vi "PVreader.vi"(2 "Device number":i8=1, 3 "VISA resource name":refnum<visa-resource-name>) -> (0 "PV value":dbl=1.0 format="%.1f")   [LabVIEW 2014]
uses:
  <vilib>/Instr/_visa.llb/VISA Configure Serial Port (Instr).vi
panel:
  out "PV from ATEC302":u32
  out "lower data":u32 format="%x"
  out "Upper data":u32 format="%x"
  out "Data from ATEC302":string
  out "Data to ATEC302":string
  out "CRC data for ATEC302":string
  out "Upper CRC Byte":u32 format="%x"
  out "Lower CRC Byte":u32 format="%x"
  out "CRC =":u16 format="%x"
  out "Data without CRC":string
  out "DN HEX":string
  out "error out":errorcluster
  # "PV read"
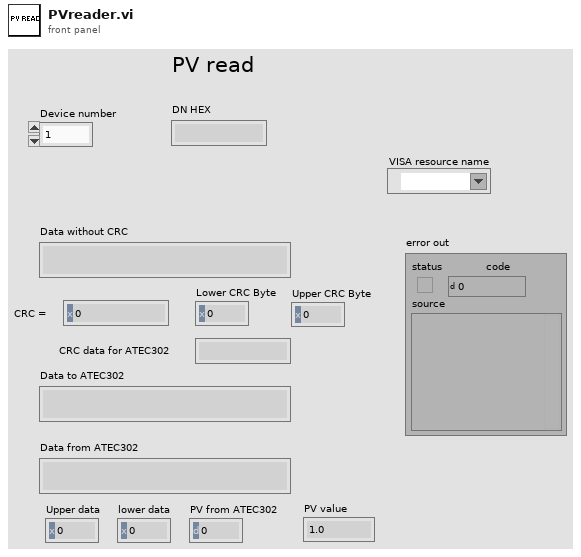
[diagram p1: front panel]
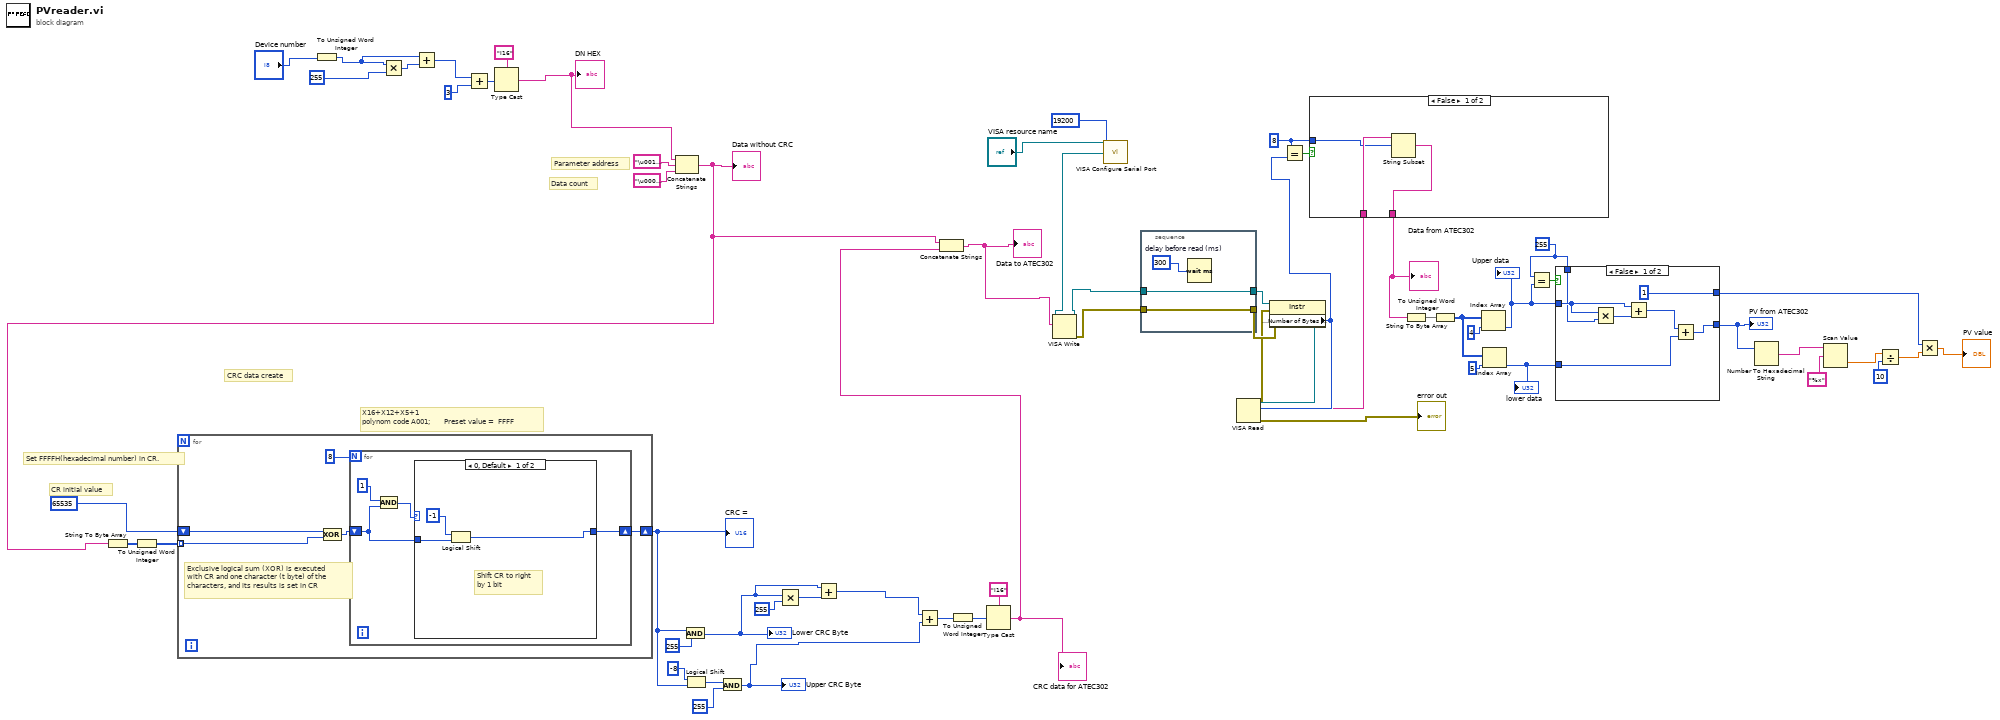
[diagram p0: block diagram]
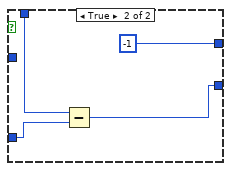
[diagram p3: hidden frame]
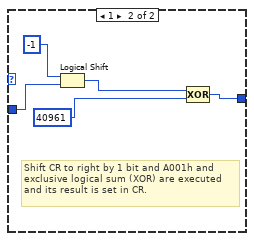
[diagram p4: hidden frame]
diagram:
  w8 = 8
  w21 = u16 255 ("y")
  # "Data count"
  # "Parameter address"
  # "CRC data create"
  # "Set FFFFH(hexadecimal number) in CR."
  # "CR initial value"
  # "X16+X12+X5+1\npolynom code A001;       Preset value =  FFFF"
  n1 = To Unsigned Word Integer(number="Device number") -> (unsigned 16bit integer=w54:u16)
  n2 = Multiply(x=w54, y=u16 255) -> (x*y=w56:u16)
  n3 = Add(x=w54, y=w56) -> (x+y=w55:u16)
  n4 = Add(x=w55, y=u16 3) -> (x+y=w57:u16)
  n5 = Type Cast(type="I16", x=w57) -> (*(type *) &x=w53:string)
  "DN HEX" <- w53
  n6 = Concatenate Strings(w53, "\u0010\u0000", "\u0000\u0001") -> (w37:string)
  "Data without CRC" <- w37
  n7 = String To Byte Array(string=w37) -> (unsigned byte array=w51:u8[])
  n8 = To Unsigned Word Integer(number=w51) -> (unsigned 16bit integer=w50:u16[])
  n9 = for {
    shift-right: [w63] -> w46
    shift-left: u16 65535 -> [w64]
    tunnel: w50 -> [w62] mode=indexing
    # "Exclusive logical sum (XOR) is executed\nwith CR and one character (t byte) of the\ncharacters, and its results is set in CR"
    n10 = Compound Arithmetic op=XOR(w64, w62) -> (w65:u32)
    n11 = for {
      N: 8 -> [_]
      shift-right: [w69] -> w63
      shift-left: w65 -> [w68]
      n12 = Compound Arithmetic op=AND(u16 1, w68) -> (w67:u32)
      n13 = case shown="0, Default" w67 {
        tunnel: [w72 w77] -> w69
        tunnel: w68 -> [w71 w74]
        frame 0, Default {
          # "Shift CR to right\nby 1 bit"
          n14 = Logical Shift(y=i16 -1, x=w71) -> (x << y=w72:u32)
        }
        frame 1 {
          # "Shift CR to right by 1 bit and A001h and\nexclusive logical sum (XOR) are executed\nand its result is set in CR."
          n15 = Logical Shift(y=i16 -1, x=w74) -> (x << y=w76:u32)
          n16 = Compound Arithmetic op=XOR(w76, u32 40961) -> (w77:u32)
        }
      }
    }
  }
  "CRC =" <- w46
  n17 = And(x=w46, y=u16 255) -> (x .and. y?=w40:u32)
  "Lower CRC Byte" <- w40
  n18 = Logical Shift(y=i16 -8, x=w46) -> (x << y=w47:u32)
  n19 = And(x=w47, y=u16 255) -> (x .and. y?=w43:u32)
  "Upper CRC Byte" <- w43
  n20 = Multiply(x=w40, y=u16 255) -> (x*y=w41:u32)
  n21 = Add(x=w40, y=w41) -> (x+y=w42:u32)
  n22 = Add(x=w42, y=w43) -> (x+y=w35:u32)
  n23 = To Unsigned Word Integer(number=w35) -> (unsigned 16bit integer=w38:u16)
  n24 = Type Cast(type="I16", x=w38) -> (*(type *) &x=w36:string)
  "CRC data for ATEC302" <- w36
  n25 = Concatenate Strings(w37, w36) -> (w4:string)
  "Data to ATEC302" <- w4
  n26 = call-poly "VISA Configure Serial Port"("VISA resource name"="VISA resource name", "baud rate (9600)"=u32 19200) -> ("VISA resource name out"=w3:refnum<visa-resource-name>)  [unwired: 12 in, 1 out]
  n27 = VISA Write(VISA resource name=w3, write buffer=w4) -> (VISA resource name out=w2:refnum<visa-resource-name>, error out=w1:errorcluster)  [unwired: 1 in, 1 out]
  n28 = stacked-sequence {
    tunnel: w1 -> [w81]
    tunnel: [w81] -> w15
    tunnel: w2 -> [w80]
    tunnel: [w80] -> w13
    frame #0 {
      w79 = u32 300  # delay before read (ms)
      n29 = Wait (ms)(milliseconds to wait=w79) -> ()  [unwired: 1 out]
    }
  }
  n30 = property class="Instr"(reference=w13, error in=w15) -> (reference out=w12:refnum<visa-resource-name>, error out=w14:errorcluster, "Serial Settings:Number of Bytes at Serial Port"=w11:u32)
  n31 = VISA Read(VISA resource name=w12, byte count=w11, error in (no error)=w14) -> (read buffer=w7:string, error out=→"error out":errorcluster)  [unwired: 2 out]
  n32 = Equal?(x=w8, y=w11) -> (x = y?=w9:bool)
  n33 = case shown="False" w9 {
    tunnel: w7 -> [w84 w85]
    tunnel: [w82 w85] -> w10
    tunnel: w8 -> [w83 _]
    frame False {
      n34 = String Subset(string=w84, offset (0)=w83) -> (substring=w82:string)  [unwired: 1 in]
    }
    frame True {
    }
  }
  "Data from ATEC302" <- w10
  n35 = String To Byte Array(string=w10) -> (unsigned byte array=w31:u8[])
  n36 = To Unsigned Word Integer(number=w31) -> (unsigned 16bit integer=w28:u16[])
  n37 = Index Array(array=w28, index=u16 4 ("y")) -> (element=w23:u16)
  "Upper data" <- w23
  n38 = Index Array(array=w28, index=u16 5 ("y")) -> (element=w17:u16)
  "lower data" <- w17
  n39 = Equal?(x=w21, y=w23) -> (x = y?=w22:bool)
  n40 = case shown="False" w22 {
    tunnel: w23 -> [w91 _]
    tunnel: w21 -> [w90 w94]
    tunnel: [1 -1] -> w20
    tunnel: w17 -> [w87 w95]
    tunnel: [w86 w93] -> w16
    frame False {
      n41 = Multiply(x=w91, y=w90) -> (x*y=w92:u16)
      n42 = Add(x=w91, y=w92) -> (x+y=w88:u16)
      n43 = Add(x=w88, y=w87) -> (x+y=w86:u16)
    }
    frame True {
      n44 = Subtract(x=w94, y=w95) -> (x-y=w93:u16)
    }
  }
  "PV from ATEC302" <- w16
  n45 = Number To Hexadecimal String(2:w16) -> (0:w24:string)  [unwired: 1 in]
  n46 = Scan Value(string=w24, format string="%x") -> (value=w25:dbl)  [unwired: 1 in, 1 out]
  n47 = Divide(x=w25, y=10) -> (x/y=w19:dbl)
  n48 = Multiply(x=w20, y=w19) -> (x*y=→"PV value":dbl)
